vi "SSL_Connect.vi"(8 "error in (no error)":errorcluster, 11 "SSL in":refnum<class "SSL.lvclass">) -> (0 "error out":errorcluster, 3 "SSL out":refnum<class "SSL.lvclass">)   [LabVIEW 2013, in "SSL_Lib.lvlib" / "SSL.lvclass"]
uses:
  SSL.lvclass
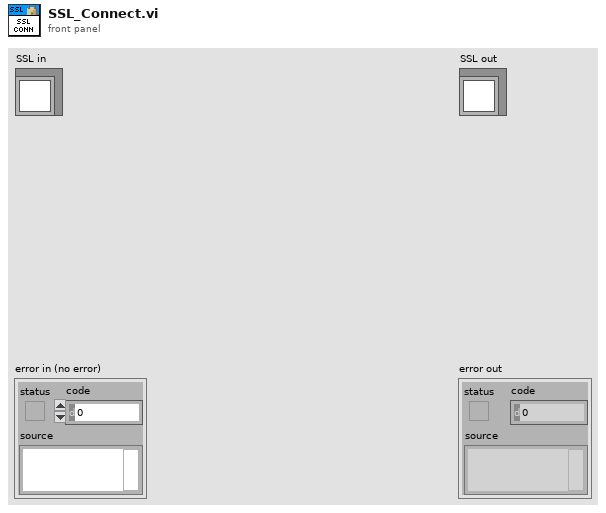
[diagram p1: front panel]
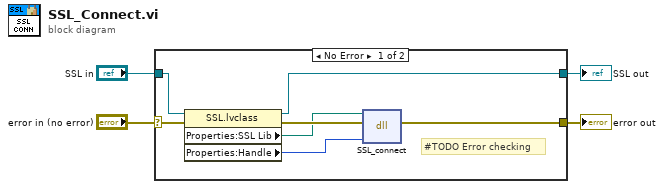
[diagram p0: block diagram]
diagram:
  n1 = case shown="No Error" "error in (no error)" {
    selector: "error in (no error)" -> [w11 w13]
    tunnel: [w10 w13] -> w3
    tunnel: [w5 w12] -> w1
    tunnel: "SSL in" -> [w8 w12]
    frame No Error {
      # "#TODO Error checking"
      n2 = property class="SSL.lvclass"(reference=w8, error in=w11) -> (reference out=w5:refnum<class "SSL.lvclass">, error out=w9:errorcluster, "Properties:SSL Lib"=w7:path, "Properties:Handle"=w6:u64)
      n3 = dll-call lib="C:/Program Files (x86)/National Instruments/Shared/nissl/NIssleay32.dll" fn="SSL_connect"(path in=w7, error in=w9, "*SSL"=w6) -> (error out=w10:errorcluster)  [unwired: 3 in, 1 out]
    }
    frame Error {
    }
  }
  "error out" <- w3
  "SSL out" <- w1
